vi "Spi Slave.vi"(0 "spi input":T3, 11 "MISO data":u64 format="%.0x", 13 "transfer settings":T2) -> (4 "spi output":T4, 6 "data output enable":bool, 8 "MOSI data":u64 format="%.0x", 10 "MOSI data valid":bool, 15 "read bit status":T1)   [LabVIEW 2013, in "NI SPI IP (FPGA).lvlib"]
doc: "This VI implements a SPI slave that is compliant with 4-wire (unidirectional input and output data) SPI transfers. \n\nPlease see the documentation included with this example for details on how to include this VI into your application."
uses:
  NI SPI IP (FPGA).lvlib
  Spi Master Inputs.ctl
  Spi Master Outputs.ctl
  Slave Transfer Settings.ctl
  Read Bit Status.ctl
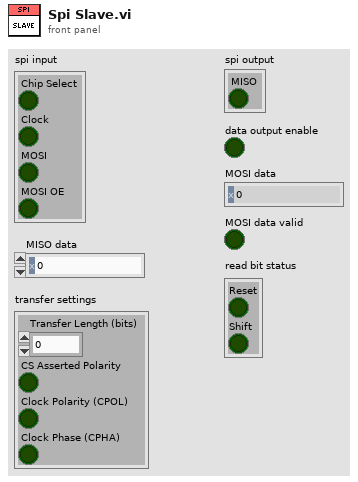
[diagram p1: front panel]
types:
  T1 = typedef "NI SPI IP (FPGA).lvlib/Read Bit Status.ctl" = cluster{"Reset":bool, "Shift":bool}
  T2 = typedef "NI SPI IP (FPGA).lvlib/Slave Transfer Settings.ctl" = cluster{"Transfer Length (bits)":u8, "CS Asserted Polarity":bool, "Clock Polarity (CPOL)":bool, "Clock Phase (CPHA)":bool}
  T3 = typedef "NI SPI IP (FPGA).lvlib/Spi Master Outputs.ctl" = cluster{"Chip Select":bool, "Clock":bool, "MOSI":bool, "MOSI OE":bool}
  T4 = typedef "NI SPI IP (FPGA).lvlib/Spi Master Inputs.ctl" = cluster{"MISO":bool}
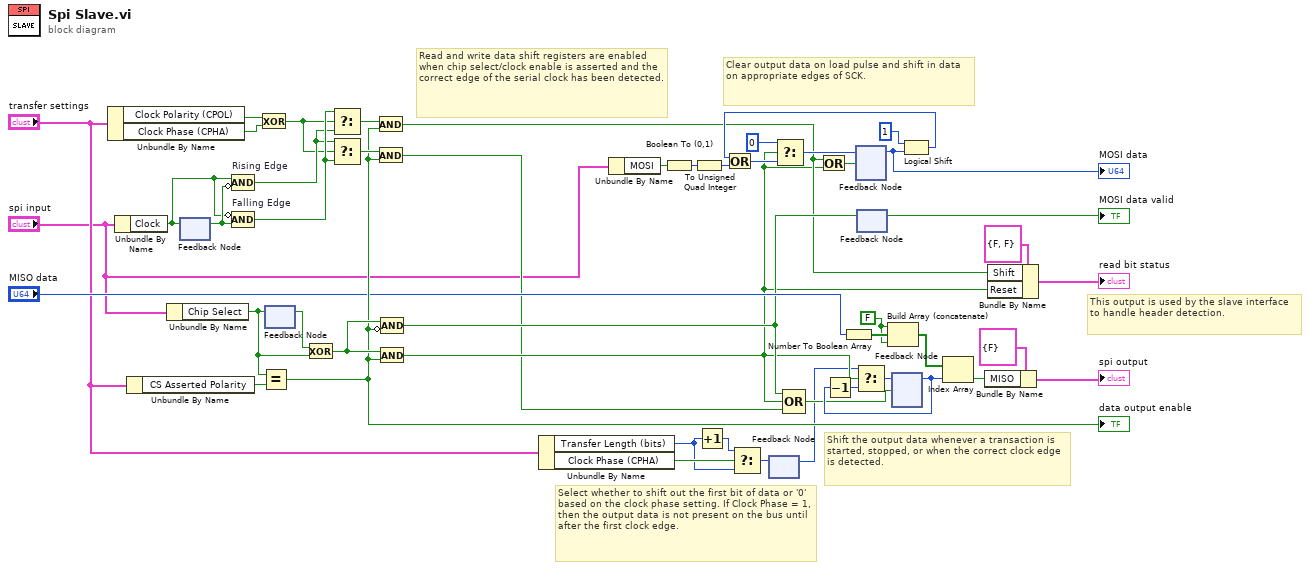
[diagram p0: block diagram]
diagram:
  w8 = FALSE
  # "This output is used by the slave interface to handle header detection."
  # "Select whether to shift out the first bit of data or '0' based on the clock phase setting. If Clock Phase = 1, then the output data is not present on the bus until after the first clock edge."
  # "Shift the output data whenever a transaction is started, stopped, or when the correct clock edge is detected."
  # "Clear output data on load pulse and shift in data on appropriate edges of SCK."
  # "Read and write data shift registers are enabled when chip select/clock enable is asserted and the correct edge of the serial clock has been detected."
  n1 = Unbundle By Name("transfer settings") -> ("Clock Polarity (CPOL)"=w30:bool, "Clock Phase (CPHA)"=w29:bool)
  n2 = Unbundle By Name("spi input") -> ("Clock"=w48:bool)
  n3 = Unbundle By Name("transfer settings") -> ("CS Asserted Polarity"=w39:bool)
  n4 = Unbundle By Name("spi input") -> ("Chip Select"=w33:bool)
  n5 = feedback-in #1(w48) -> ()
  n6 = feedback #1() -> (w49:bool)  [unwired: 1 in]
  n7 = Compound Arithmetic op=AND "Rising Edge"(w48, invert w49) -> (w27:bool)
  n8 = Compound Arithmetic op=AND "Falling Edge"(invert w48, w49) -> (w28:bool)
  n9 = Exclusive Or(1:w29, 2:w30) -> (0:w26:bool)
  n10 = Equal?(x=w33, y=w39) -> (x = y?=w24:bool)
  "data output enable" <- w24
  n11 = feedback #2() -> (w40:bool)  [unwired: 1 in]
  n12 = feedback-in #2(w33) -> ()
  n13 = Exclusive Or(1:w33, 2:w40) -> (0:w25:bool)
  n14 = Select(t=w28, s=w26, f=w27) -> (s? t:f=w31:bool)
  n15 = Select(t=w27, s=w26, f=w28) -> (s? t:f=w32:bool)
  n16 = And(x=w31, y=w24) -> (x .and. y?=w12:bool)
  n17 = And(x=w32, y=w24) -> (x .and. y?=w3:bool)
  n18 = And(x=w25, y=w24) -> (x .and. y?=w11:bool)
  n19 = Compound Arithmetic op=AND(w25, invert w24) -> (w15:bool)
  n20 = Unbundle By Name("transfer settings") -> ("Transfer Length (bits)"=w6:u8, "Clock Phase (CPHA)"=w9:bool)
  n21 = Unbundle By Name("spi input") -> ("MOSI"=w34:bool)
  n22 = Boolean To (0,1)(Boolean=w34) -> (0, 1=w45:i16)
  n23 = To Unsigned Quad Integer(1:w45) -> (0:w43:u64)
  n24 = Increment(x=w6) -> (x+1=w7:u8)
  n25 = Select(t=w7, s=w9, f=w6) -> (s? t:f=w5:u8)
  n26 = feedback #3() -> (w4:u8)  [unwired: 1 in]
  n27 = feedback-in #3(w5) -> ()
  n28 = Compound Arithmetic op=OR(w15, w11, w3) -> (w14:bool)
  n29 = Or(x=w12, y=w11) -> (x .or. y?=w38:bool)
  n30 = Number To Boolean Array(number="MISO data") -> (Boolean array=w20:bool[])
  n31 = feedback #4() -> (w47:u64)  [unwired: 1 in]
  "MOSI data" <- w47
  n32 = feedback-in #5(w15) -> ()
  n33 = feedback #5() -> (→"MOSI data valid":bool)  [unwired: 1 in]
  n34 = Build Array (concatenate)(w8, w20, w8) -> (w19:bool[])
  n35 = feedback #6() -> (w17:u8)  [unwired: 1 in]
  n36 = Decrement(x=w17) -> (x-1=w16:u8)
  n37 = Select(t=w4, s=w11, f=w16) -> (s? t:f=w18:u8)
  n38 = feedback-in #6(w18, w14) -> ()
  n39 = Logical Shift(y=i8 1, x=w47) -> (x << y=w44:u64)
  n40 = Or(x=w44, y=w43) -> (x .or. y?=w37:u64)
  n41 = Select(t=u64 0, s=w11, f=w37) -> (s? t:f=w36:u64)
  n42 = feedback-in #4(w36, w38) -> ()
  n43 = Index Array(array=w19, index=w17) -> (element=w21:bool)
  n44 = Bundle By Name(cluster=T4 {"MISO"=FALSE} ("SPI.Output"), "MISO"=w21) -> (→"spi output":T4)
  n45 = Bundle By Name(cluster=T1 {"Reset"=FALSE, "Shift"=FALSE} ("ReadBitStatus"), "Shift"=w12, "Reset"=w11) -> (→"read bit status":T1)
